vi "Create ZIP Archive.vi"(10 "Source File/Directory":path, 11 "Target Zip File":path) -> (0 "error out":errorcluster, 3 "Path to .zip":path)   [LabVIEW 2011]
doc: "This VI will zip-up a Source File or Directory into the Target Zip File.\n\nInstructions:\n1) Run the VI\n2) Select a zip file that you want to create or overwrite (Target Zip File).\n3) Select either a file or directory that you want to compress (Source File/Directory)."
panel:
  out "In Progress":bool
  out "Directory Tree":string(tree)
  # "This VI will zip-up a Source File or Directory into the Target Zip File.\n\nInstructions:\n1) Run the VI\n2) Select a zip file that you want to create or overwrite (Target Zip File).\n3) Select either a file or directory that you want to compress (Source File/Directory)."
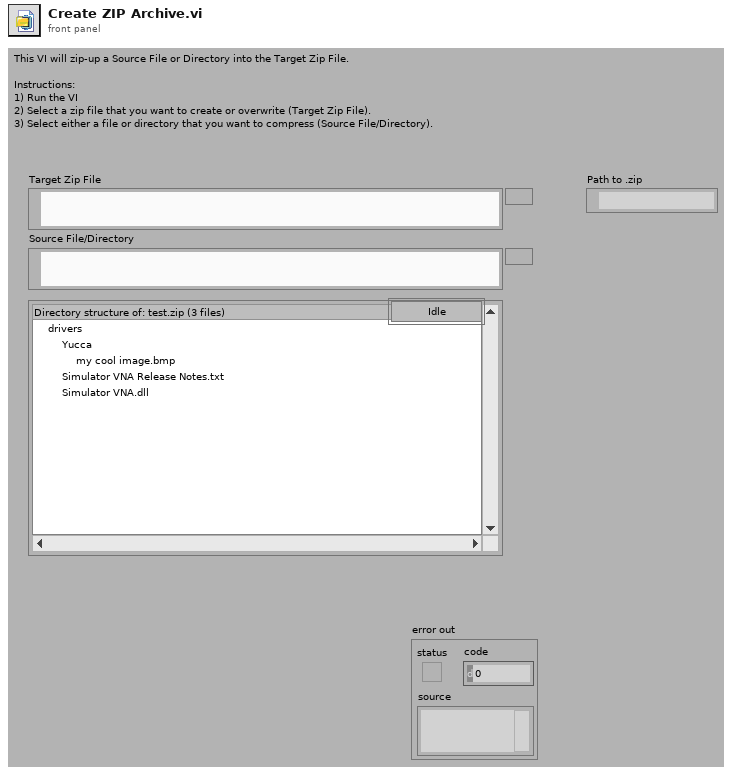
[diagram p1: front panel]
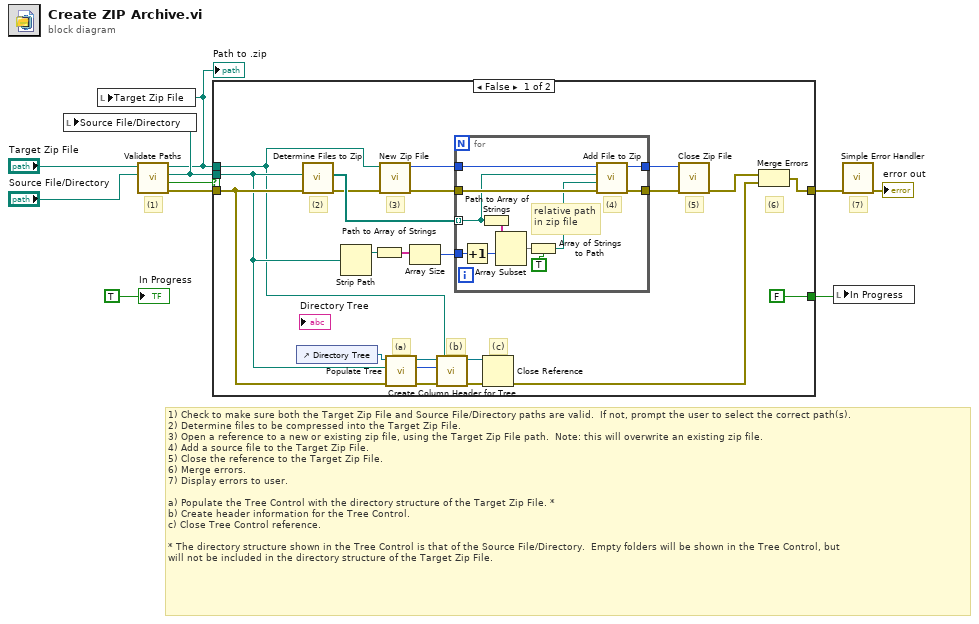
[diagram p0: block diagram]
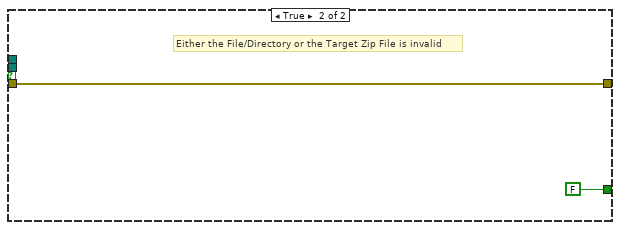
[diagram p2: hidden frame]
diagram:
  # "(7)"
  # "1) Check to make sure both the Target Zip File and Source File/Directory paths are valid.  If not, prompt the user to select the correct path(s).\n2) Determine files to be compressed into the Target Zip File.\n3) Open a reference to a new or existing zip file, using the Target Zip File path.  Note: this will overwrite an existing zip file.\n4) Add a source file to the Target Zip File.\n5) Close the reference to the Target Zip File.\n6) Merge errors.\n7) Display errors to user.\n\na) Populate the Tree Control with the directory structure of the Target Zip File. *\nb) Create header information for the Tree Control.\nc) Close Tree Control reference.\n\n* The directory structure shown in the Tree Control is that of the Source File/Directory.  Empty folders will be shown in the Tree Control, but \nwill not be included in the directory structure of the Target Zip File."
  # "(1)"
  n1 = call "Validate Paths.vi"("File or Directory input"="Source File/Directory", "Target zip file input"="Target Zip File") -> ("error out"=w6:errorcluster, "Invalid Path?"=w7:bool, "File or Directory selected"=w5:path, "Target zip file selected"=w1:path)  [unwired: 6 out]
  "Path to .zip" <- w1
  n2 = local write "Source File/Directory"(w5) -> ()
  n3 = local write "Target Zip File"(w1) -> ()
  n4 = case shown="False" w7 {
    tunnel: w5 -> [w13 _]
    tunnel: [w23 w45] -> w9
    tunnel: w6 -> [w22 w45]
    tunnel: w1 -> [w12 _]
    tunnel: [FALSE ("In Progress") FALSE ("In Progress")] -> w3
    frame False {
      # "(6)"
      # "(c)"
      # "(b)"
      # "(a)"
      # "(5)"
      # "(3)"
      # "(2)"
      n5 = control-ref of="Directory Tree"() -> (w19:refnum<vi>)
      n6 = call "Determine Files to Zip.vi"("error in (no error)"=w22, "File or Directory"=w13) -> ("error out"=w21:errorcluster, "Array"=w27:path[])  [unwired: 8 out]
      n7 = Strip Path(path=w13) -> (stripped path=w30:path)  [unwired: 1 out]
      n8 = Path to Array of Strings(0:w30) -> (2:w29:string[])  [unwired: 1 out]
      n9 = call <vilib>:"New Zip File.vi"("error in (no error)"=w21, "target"=w12) -> ("error out"=w31:errorcluster, "zip file out"=w32:i64)  [unwired: 1 in, 3 out]
      n10 = call "Populate Tree.vi"("error in (no error)"=w22, "File or Directory"=w13, "Directory Tree"=w19) -> ("error out"=w20:errorcluster, "Number of files found"=w17:i32, "Directory Tree dup"=w18:refnum<vi>)  [unwired: 6 out]
      n11 = Array Size(array=w29) -> (size(s)=w28:i32)
      n12 = call "Create Column Header for Tree.vi"("Target zip file"=w12, "error in (no error)"=w20, "Number of Files Found"=w17, "Directory Tree"=w18) -> ("error out"=w15:errorcluster, "Directory Tree dup"=w16:refnum<vi>)  [unwired: 2 in, 4 out]
      n13 = for {
        tunnel: w27 -> [w41] mode=indexing
        tunnel: w32 -> [w43]
        tunnel: w31 -> [w42]
        tunnel: w28 -> [w39]
        tunnel: [w35] -> w26
        tunnel: [w34] -> w25
        # "(4)"
        # "relative path\nin zip file"
        n14 = Increment(x=w39) -> (x+1=w33:i32)
        n15 = Path to Array of Strings(0:w41) -> (2:w40:string[])  [unwired: 1 out]
        n16 = Array Subset(array=w40, index=w33) -> (w38:string[])  [unwired: 1 in]
        n17 = Array of Strings to Path(0:w38, 1:TRUE ("relative")) -> (2:w37:path)
        n18 = call <vilib>:"Add File to Zip.vi"("error in (no error)"=w42, "destination path in zip"=w37, "source file path"=w41, "zip file in"=w43) -> ("error out"=w35:errorcluster, "zip file out"=w34:i64)  [unwired: 6 out]
      }
      n19 = Close Reference(reference=w16, error in (no error)=w15) -> (error out=w14:errorcluster)
      n20 = call <vilib>:"Close Zip File.vi"("error in (no error)"=w26, "zip file in"=w25) -> ("error out"=w24:errorcluster)  [unwired: 1 in, 4 out]
      n21 = Merge Errors(w24, w14) -> (w23:errorcluster)
    }
    frame True {
      # "Either the File/Directory or the Target Zip File is invalid"
    }
  }
  n22 = local write "In Progress"(w3) -> ()
  n23 = call <vilib>:"Simple Error Handler.vi"("error in (no error)"=w9) -> ("error out"=→"error out":errorcluster)  [unwired: 1 in, 7 out]
  "In Progress" <- TRUE ("In Progress")
